vi "CRYSet Enable Disable for Run.vi"(0 "sOption":string="Move Up") -> ()   [LabVIEW 2013]
uses:
  CRYProject/CRYProject Editor Global.vi
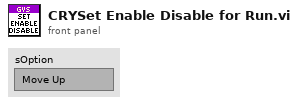
[diagram p1: front panel]
types:
  T1 = enum8{"Enabled", "Disabled", "Disabled and Grayed Out"}
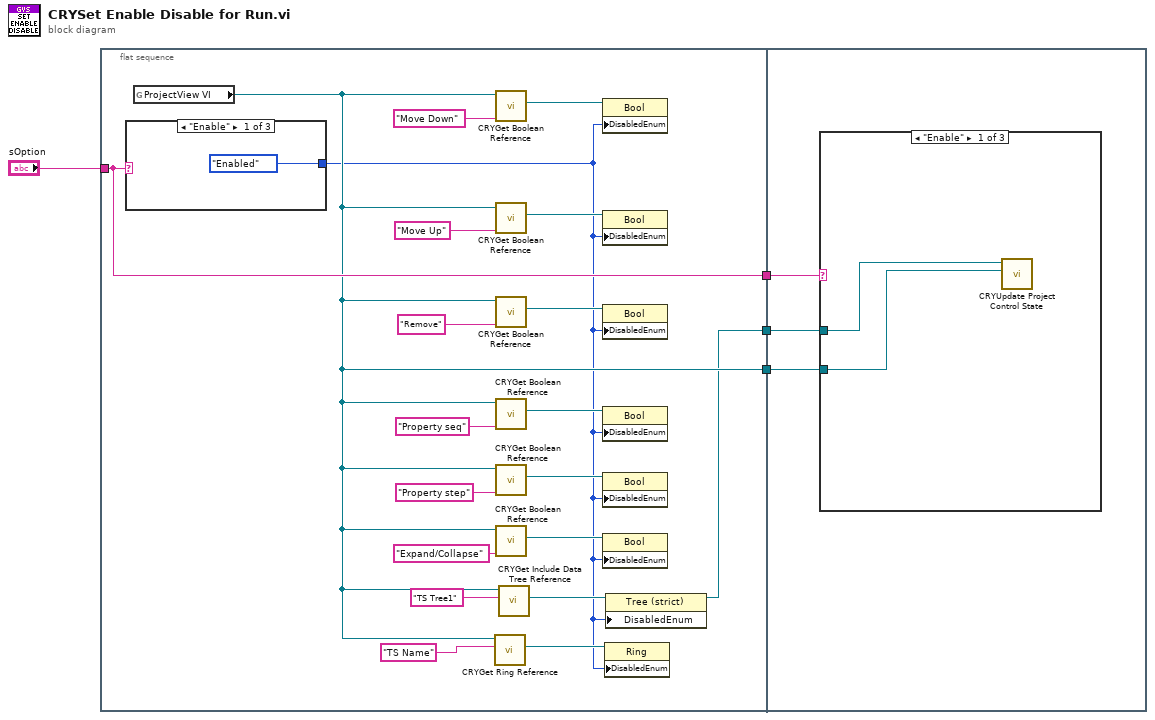
[diagram p0: block diagram]
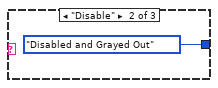
[diagram p2: hidden frame]
diagram:
  n1 = flat-sequence {
    tunnel: "sOption" -> [w8]
    tunnel: [w8] -> w3
    tunnel: [w7] -> w2
    tunnel: [w6] -> w1
    tunnel: w3 -> [w29]
    tunnel: w2 -> [w28]
    tunnel: w1 -> [w27]
    frame #0 {
      n2 = case shown="\"Enable\"" w8 {
        tunnel: [T1."Enabled" ("Disabled") T1."Disabled and Grayed Out" ("Disabled") _] -> w5
        frame "Enable" {
        }
        frame "Disable" {
        }
        frame Default {
        }
      }
      n3 = global read "CRYProject Editor Global.vi" "ProjectView VI"() -> (w7:refnum<vi>)
      n4 = call "CRYGet Ring Reference.vi"("Label Name"="TS Name", "VI Refnum"=w7) -> ("Ring Ref Out"=w9:refnum<vi>)  [unwired: 7 in, 2 out]
      n5 = call "CRYGet Boolean Reference.vi"("Label Name"="Move Down", "VI Refnum"=w7) -> ("Boolean Ref"=w24:refnum<vi>)  [unwired: 9 out]
      n6 = call "CRYGet Boolean Reference.vi"("Label Name"="Move Up", "VI Refnum"=w7) -> ("Boolean Ref"=w22:refnum<vi>)  [unwired: 9 out]
      n7 = call "CRYGet Boolean Reference.vi"("Label Name"="Remove", "VI Refnum"=w7) -> ("Boolean Ref"=w21:refnum<vi>)  [unwired: 9 out]
      n8 = call "CRYGet Boolean Reference.vi"("Label Name"="Property seq", "VI Refnum"=w7) -> ("Boolean Ref"=w20:refnum<vi>)  [unwired: 9 out]
      n9 = call "CRYGet Boolean Reference.vi"("Label Name"="Property step", "VI Refnum"=w7) -> ("Boolean Ref"=w19:refnum<vi>)  [unwired: 9 out]
      n10 = call "CRYGet Boolean Reference.vi"("Label Name"="Expand/Collapse", "VI Refnum"=w7) -> ("Boolean Ref"=w18:refnum<vi>)  [unwired: 9 out]
      n11 = call "CRYGet Include Data Tree Reference.vi"("Label Name"="TS Tree1", "VI Refnum"=w7) -> ("Tree Ref Out"=w11:refnum<vi>)  [unwired: 7 in, 2 out]
      n12 = property class="Bool"(reference=w24, "DisabledEnum"=w5) -> ()  [unwired: 1 in, 2 out]
      n13 = property class="Bool"(reference=w22, "DisabledEnum"=w5) -> ()  [unwired: 1 in, 2 out]
      n14 = property class="Bool"(reference=w21, "DisabledEnum"=w5) -> ()  [unwired: 1 in, 2 out]
      n15 = property class="Bool"(reference=w20, "DisabledEnum"=w5) -> ()  [unwired: 1 in, 2 out]
      n16 = property class="Bool"(reference=w19, "DisabledEnum"=w5) -> ()  [unwired: 1 in, 2 out]
      n17 = property class="Bool"(reference=w18, "DisabledEnum"=w5) -> ()  [unwired: 1 in, 2 out]
      n18 = property class="Ring"(reference=w9, "DisabledEnum"=w5) -> ()  [unwired: 1 in, 2 out]
      n19 = property class="Tree (strict)"(reference=w11, "DisabledEnum"=w5) -> (reference out=w6:refnum<vi>)  [unwired: 1 in, 1 out]
    }
    frame #1 {
      n20 = case shown="\"Enable\"" w29 {
        tunnel: w28 -> [w31 _ _]
        tunnel: w27 -> [w30 _ _]
        frame "Enable" {
          n21 = call "CRYUpdate Project Control State.vi"("VI Ref"=w31, "RefTree In"=w30) -> ()  [unwired: 8 in, 2 out]
        }
        frame "Disable" {
        }
        frame Default {
        }
      }
    }
  }
